vi "Configure Hardware.vi"(8 "error in (no error)":errorcluster, 9 "Trigger Settings":T1={"Trigger Type"=enum."No Trigger", "Digital Start"={"Source"="", "Digital Start Trigger Edge"=10280}, "Digital Pause"={"Source"="", "Digital Pause Trigger Pause When"=10192}, "Digital Reference"={"Source"="", "Digital Start Trigger Edge"=10280, "Digital Reference Pretrigger Samples"=0}, "Analog Start"={"Source"="", "Analog Slope"=10280, "Analog Start Trigger Hysteresis"=0.0, "Analog Start Trigger Level"=0.0}, "Analog Pause"={"Source"="", "Analog Start Trigger Level"=0.0, "Analog Pause Trigger Pause When"=10093}, "Analog Reference"={"Source"="", "Slope"=10280, "Pretrigger Samples"=0, "Level"=0.0}, "Time Start"={"Select Time\nManually"=FALSE, "When"=timestamp(0 s since 1904-01-01)}} caption="Some parts are hidden" {"Time Start"."When" format="%<%x %.3X>T"; "Analog Reference"."Level" format="%0.2f"; "Analog Reference"."Slope" items=["Rising"=10280, "Falling"=10171]; "Analog Pause"."Analog Pause Trigger Pause When" items=["Above Level"=10093, "Below Level"=10107]; "Analog Pause"."Analog Start Trigger Level" format="%0.2f"; "Analog Start"."Analog Start Trigger Level" format="%0.2f"; "Analog Start"."Analog Start Trigger Hysteresis" format="%.2f"; "Analog Start"."Analog Slope" items=["Rising"=10280, "Falling"=10171]; "Digital Reference"."Digital Start Trigger Edge" items=["Rising"=10280, "Falling"=10171]; "Digital Pause"."Digital Pause Trigger Pause When" items=["High"=10192, "Low"=10214]; "Digital Start"."Digital Start Trigger Edge" items=["Rising"=10280, "Falling"=10171]}, 10 "DAQmx Timing Settings In":T2={"rate"=1000.0, "source"="OnboardClock", "sample mode"=10178, "samples per channel"=1000} {"sample mode" items=["Finite Samples"=10178, "Continuous Samples"=10123, "Hardware Timed Single Point"=12522]; "rate" format="%0.2f"}, 11 "HW Refnum In":string) -> (0 "error out":errorcluster, 1 "Trigger Settings Out":T1={"Trigger Type"=enum."No Trigger", "Digital Start"={"Source"="", "Digital Start Trigger Edge"=10280}, "Digital Pause"={"Source"="", "Digital Pause Trigger Pause When"=10192}, "Digital Reference"={"Source"="", "Digital Start Trigger Edge"=10280, "Digital Reference Pretrigger Samples"=0}, "Analog Start"={"Source"="", "Analog Slope"=10280, "Analog Start Trigger Hysteresis"=0.0, "Analog Start Trigger Level"=0.0}, "Analog Pause"={"Source"="", "Analog Start Trigger Level"=0.0, "Analog Pause Trigger Pause When"=10093}, "Analog Reference"={"Source"="", "Slope"=10280, "Pretrigger Samples"=0, "Level"=0.0}, "Time Start"={"Select Time\nManually"=FALSE, "When"=timestamp(0 s since 1904-01-01)}} caption="Some parts are hidden" {"Time Start"."When" format="%<%x %.3X>T"; "Analog Reference"."Level" format="%0.2f"; "Analog Reference"."Slope" items=["Rising"=10280, "Falling"=10171]; "Analog Pause"."Analog Pause Trigger Pause When" items=["Above Level"=10093, "Below Level"=10107]; "Analog Pause"."Analog Start Trigger Level" format="%0.2f"; "Analog Start"."Analog Start Trigger Level" format="%0.2f"; "Analog Start"."Analog Start Trigger Hysteresis" format="%.2f"; "Analog Start"."Analog Slope" items=["Rising"=10280, "Falling"=10171]; "Digital Reference"."Digital Start Trigger Edge" items=["Rising"=10280, "Falling"=10171]; "Digital Pause"."Digital Pause Trigger Pause When" items=["High"=10192, "Low"=10214]; "Digital Start"."Digital Start Trigger Edge" items=["Rising"=10280, "Falling"=10171]}, 2 "DAQmx Timing Settings Out":T2={"rate"=1000.0, "source"="OnboardClock", "sample mode"=10178, "samples per channel"=1000} {"sample mode" items=["Finite Samples"=10178, "Continuous Samples"=10123, "Hardware Timed Single Point"=12522]; "rate" format="%0.2f"}, 3 "HW Refnum Out":string="myvolttask")   [LabVIEW 2020, in "Acquisition.lvlib"]
doc: "Configure the hardware.\n_____\nBased on DQMH Project Template 6.0.0.91."
uses:
  Acquisition.lvlib
  Settings Editor/DAQmx Timing--cluster.ctl
  Settings Editor/DAQmx Trigger Settings--cluster.ctl
  Settings Editor/Settings Editor.lvlib
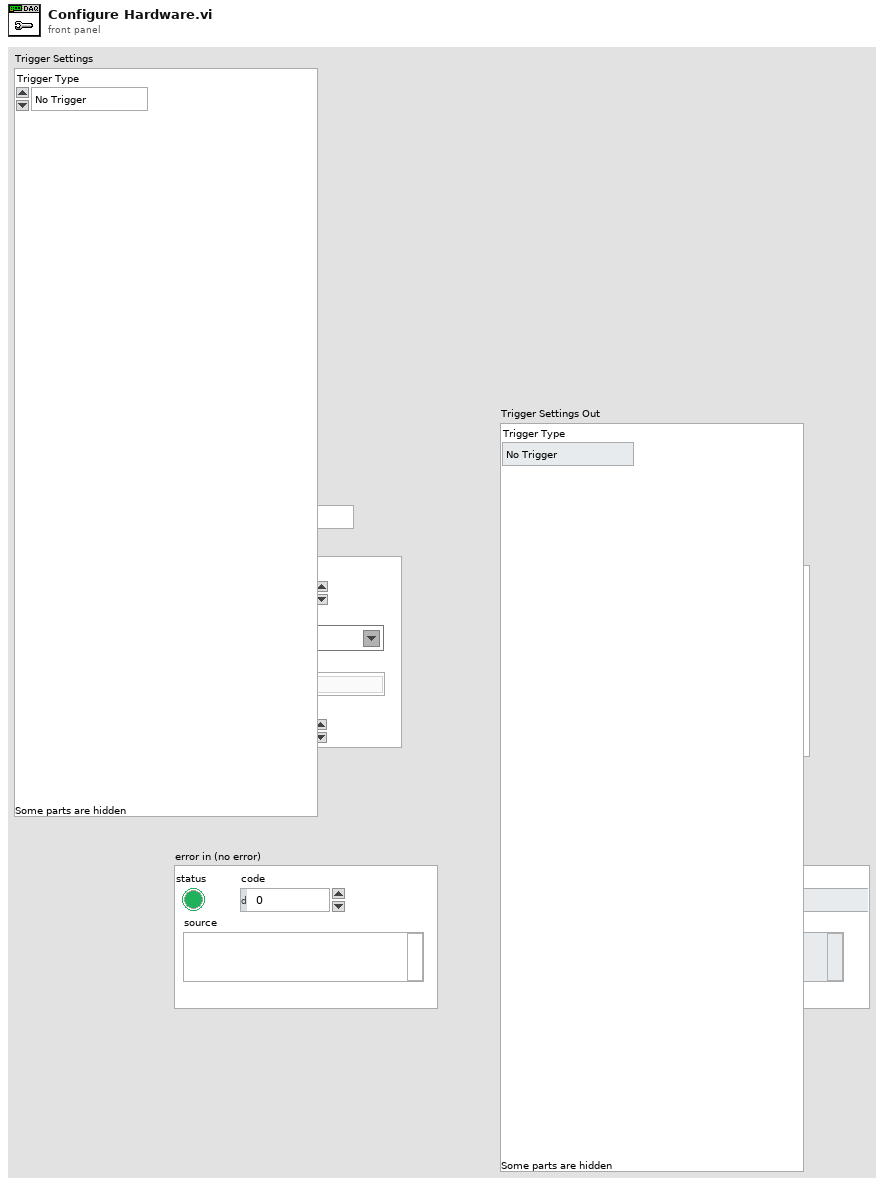
[diagram p1: front panel]
types:
  T1 = typedef "Settings Editor.lvlib/DAQmx Trigger Settings--cluster.ctl" = cluster{"Trigger Type":enum32{"No Trigger", "Digital Start", "Digital Pause", "Digital Reference", "Analog Start", "Analog Pause", "Analog Reference", "Time Start"}, "Digital Start":cluster{"Source":tag, "Digital Start Trigger Edge":i32}, "Digital Pause":cluster{"Source":tag, "Digital Pause Trigger Pause When":i32}, "Digital Reference":cluster{"Source":tag, "Digital Start Trigger Edge":i32, "Digital Reference Pretrigger Samples":u32}, "Analog Start":cluster{"Source":string, "Analog Slope":i32, "Analog Start Trigger Hysteresis":dbl, "Analog Start Trigger Level":dbl}, "Analog Pause":cluster{"Source":string, "Analog Start Trigger Level":dbl, "Analog Pause Trigger Pause When":i32}, "Analog Reference":cluster{"Source":string, "Slope":i32, "Pretrigger Samples":u32, "Level":dbl}, "Time Start":cluster{"Select Time\nManually":bool, "When":timestamp}}
  T2 = typedef "Settings Editor.lvlib/DAQmx Timing--cluster.ctl" = cluster{"rate":dbl, "source":tag, "sample mode":i32, "samples per channel":i32}
  T3 = cluster{"rate":dbl, "source":tag, "sample mode":i32, "samples per channel":i32}
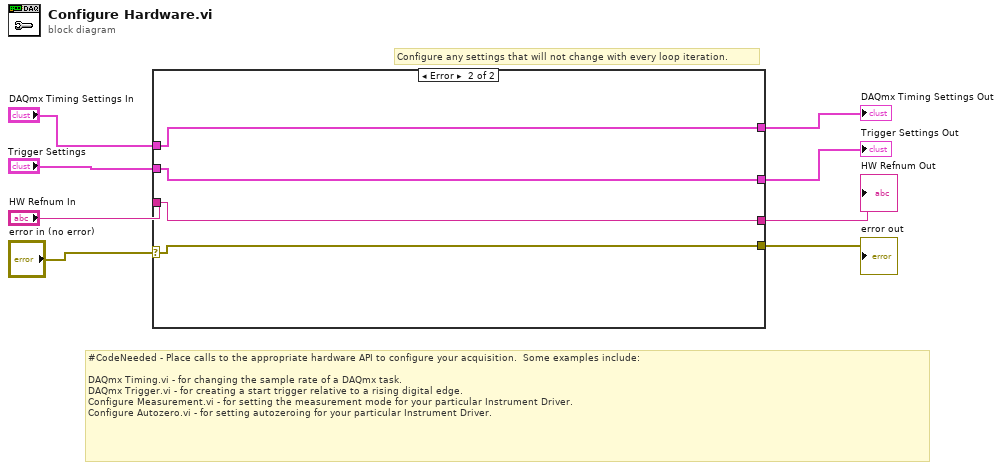
[diagram p0: block diagram]
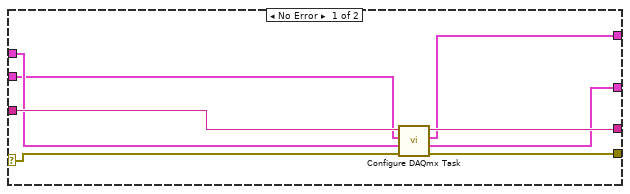
[diagram p2: hidden frame]
diagram:
  # "Configure any settings that will not change with every loop iteration."
  # "#CodeNeeded - Place calls to the appropriate hardware API to configure your acquisition.  Some examples include:\n\nDAQmx Timing.vi - for changing the sample rate of a DAQmx task.\nDAQmx Trigger.vi - for creating a start trigger relative to a rising digital edge.\nConfigure Measurement.vi - for setting the measurement mode for your particular Instrument Driver.\nConfigure Autozero.vi - for setting autozeroing for your particular Instrument Driver."
  n1 = case shown="Error" "error in (no error)" {
    selector: "error in (no error)" -> [w15 w19]
    tunnel: [w14 w19] -> w4
    tunnel: "HW Refnum In" -> [w16 w20]
    tunnel: [w13 w20] -> w7
    tunnel: "DAQmx Timing Settings In" -> [w12 w18]
    tunnel: "Trigger Settings" -> [w11 w17]
    tunnel: [w10 w18] -> w2
    tunnel: [w9 w17] -> w1
    frame No Error {
      n2 = call "Configure DAQmx Task.vi"("error in (no error)"=w15, "DAQmx Timing Settings In"=w12, "Trigger Settings In"=w11, "HW Refnum In"=w16) -> ("error out"=w14:errorcluster, "Trigger Settings Out"=w9:T1, "DAQmx Timing Settings Out"=w10:T3, "HW Refnum Out"=w13:string)  [unwired: 4 in]
    }
    frame Error {
    }
  }
  "error out" <- w4
  "HW Refnum Out" <- w7
  "Trigger Settings Out" <- w1
  "DAQmx Timing Settings Out" <- w2
